vi "filter.vi"(0 "Image In":T2, 1 "Red BCG Values (Brightness 1)":T1={"Brightness"=142.42021, "Contrast"=69.80851, "Gamma"=2.51808}, 2 "Green BCG Values (Brightness 1)":T1={"Brightness"=142.42021, "Contrast"=69.80851, "Gamma"=2.51808}, 3 "Blue BCG Values (Brightness 1)":T1={"Brightness"=142.42021, "Contrast"=69.80851, "Gamma"=2.51808}, 4 "Range (Threshold 1)":cluster{"Lower value":sgl, "Upper value":sgl}={"Lower value"=109.28571, "Upper value"=255.0}, 7 "error in":errorcluster) -> (20 "Image Out":T2, 21 "Number of Particles (Particle Analysis 1)":i32, 22 "Particle Measurements (Pixels) (Particle Analysis 1)":dbl[][](array[numeric]) format="%.2f", 23 "Particle Measurements (Real-World) (Particle Analysis 1)":dbl[][](array[numeric]) format="%.2f", 27 "error out":errorcluster)   [LabVIEW 2020]
uses:
  <vilib>/vision/Image Controls.llb/IMAQ Image.ctl
  <vilib>/vision/NI_Vision_Development_Module.lvlib
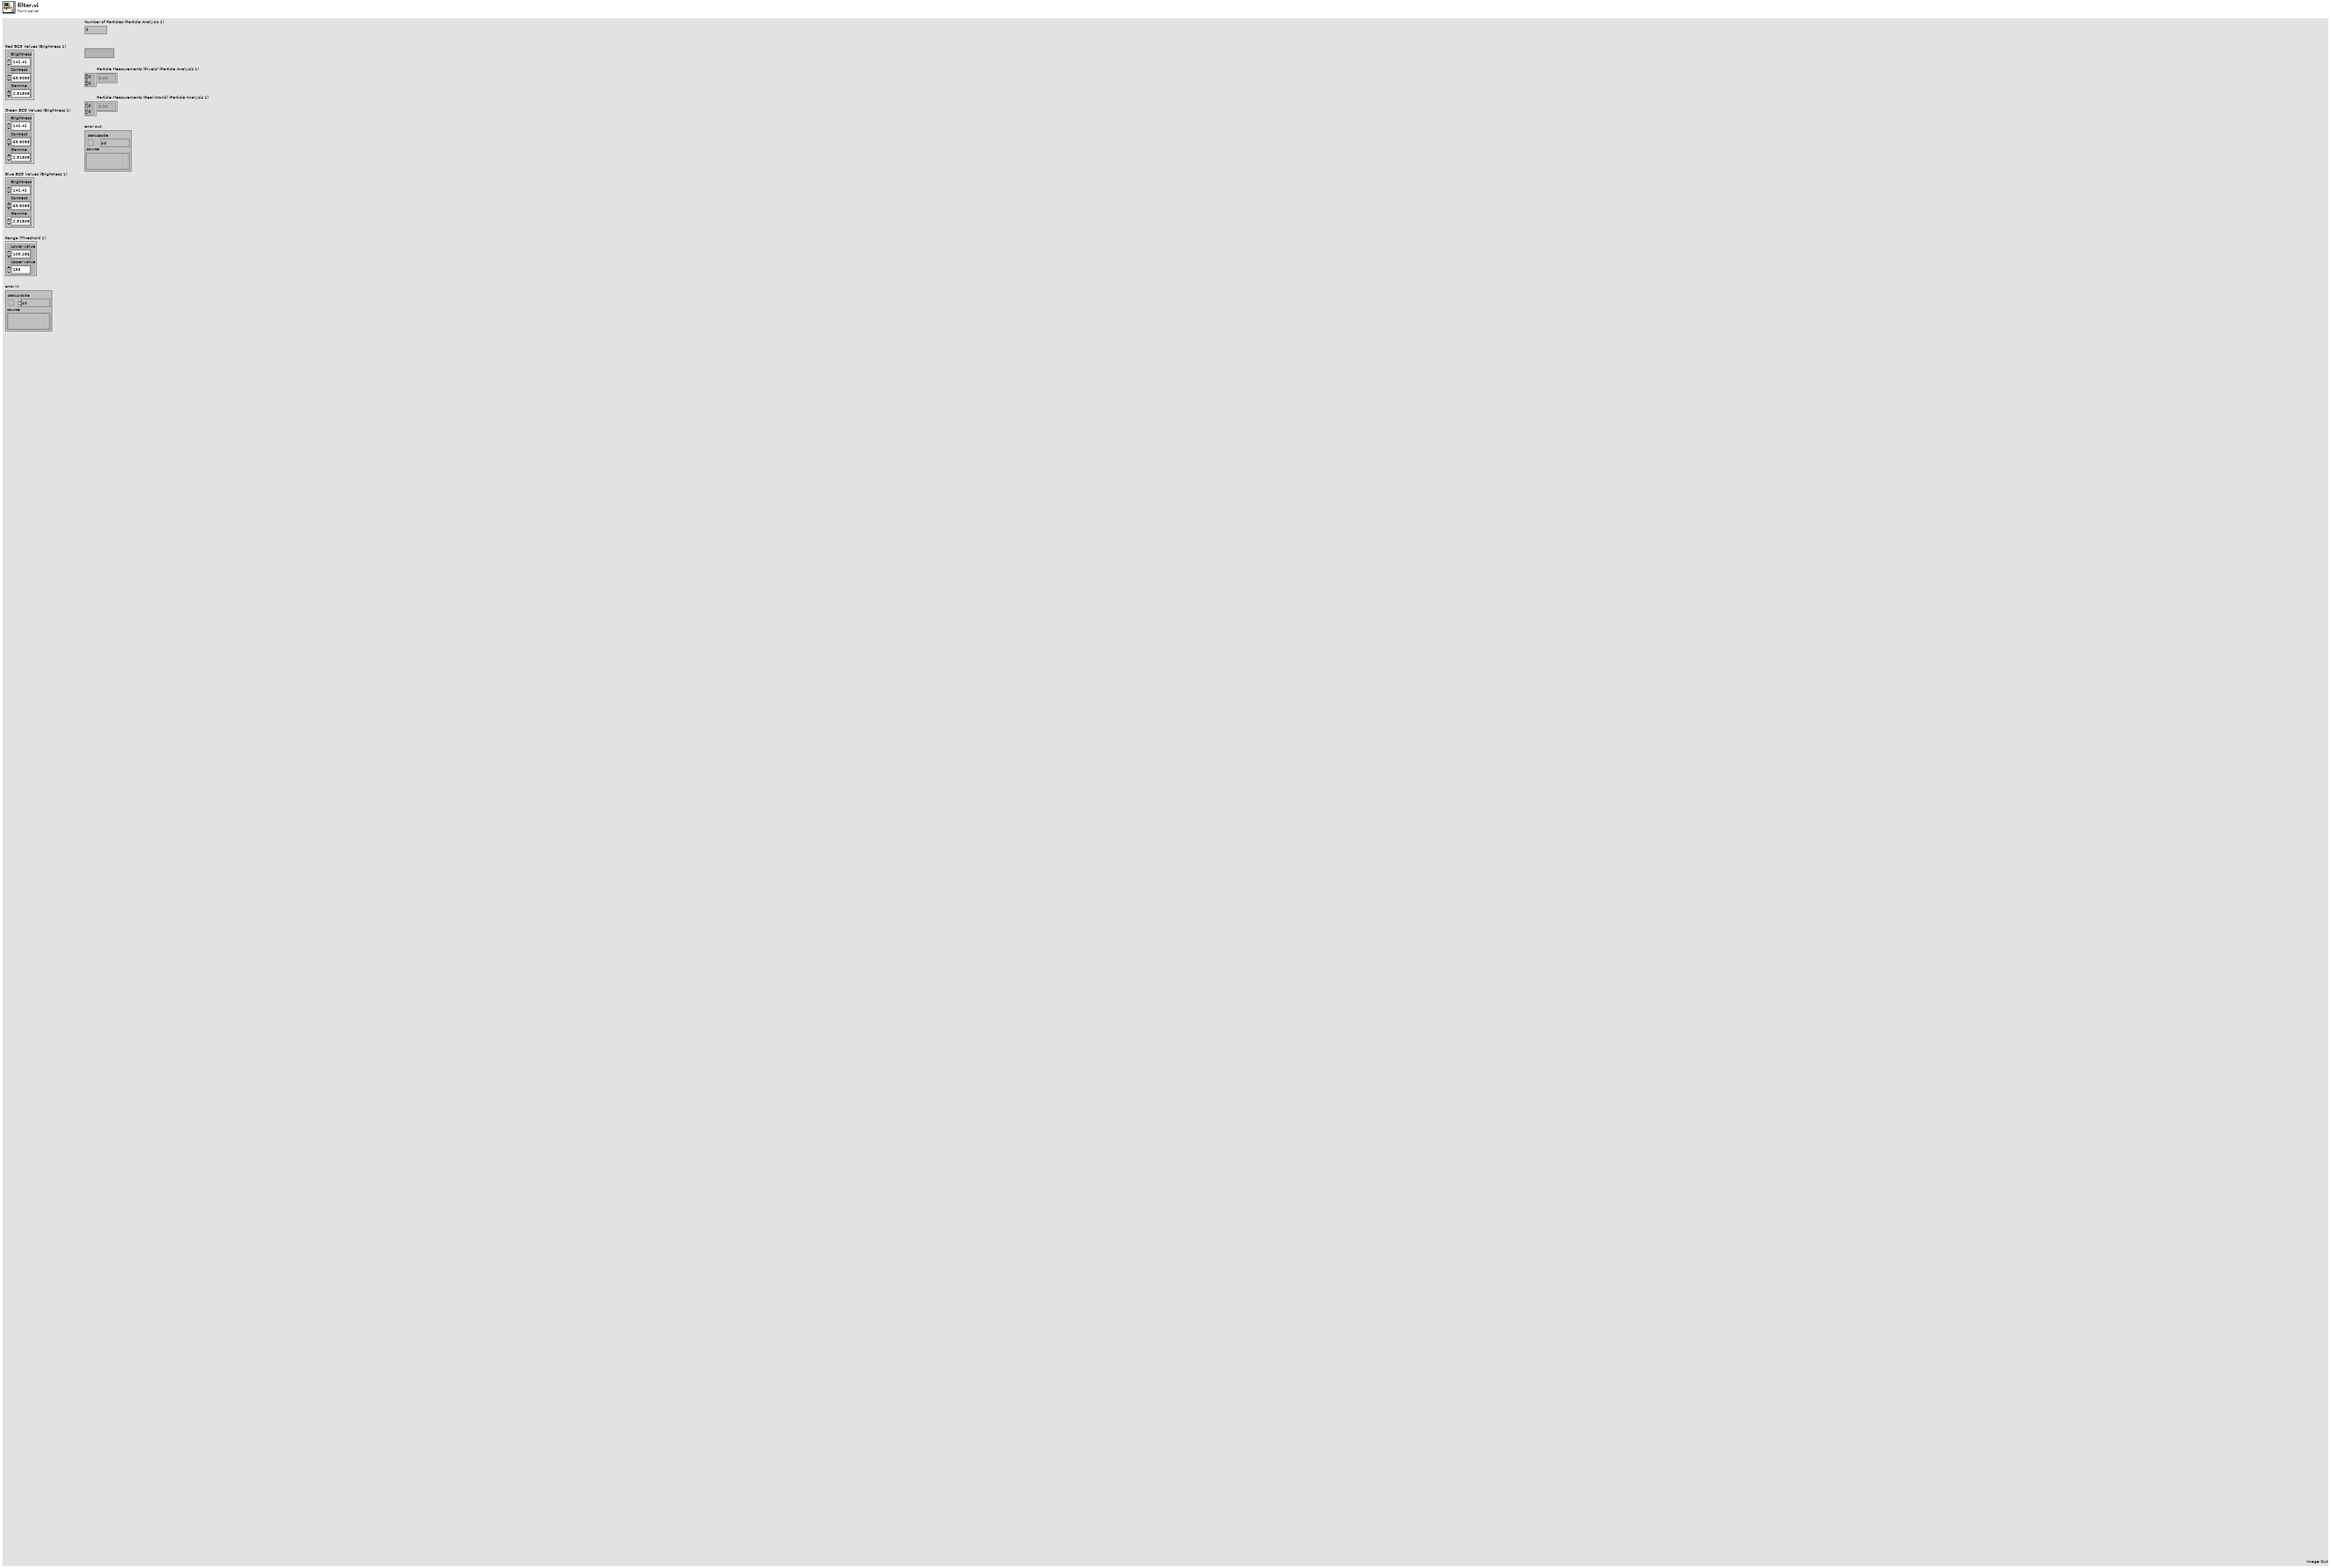
[diagram p1: front panel]
types:
  T1 = cluster{"Brightness":sgl, "Contrast":sgl, "Gamma":sgl}
  T2 = typedef "IMAQ Image.ctl" = refnum<image>
  T3 = cluster{"Measurement Parameter":i32, "Range Lower Value":dbl, "Range Upper Value":dbl, "Range":bool, "Measurement Type":bool}[]
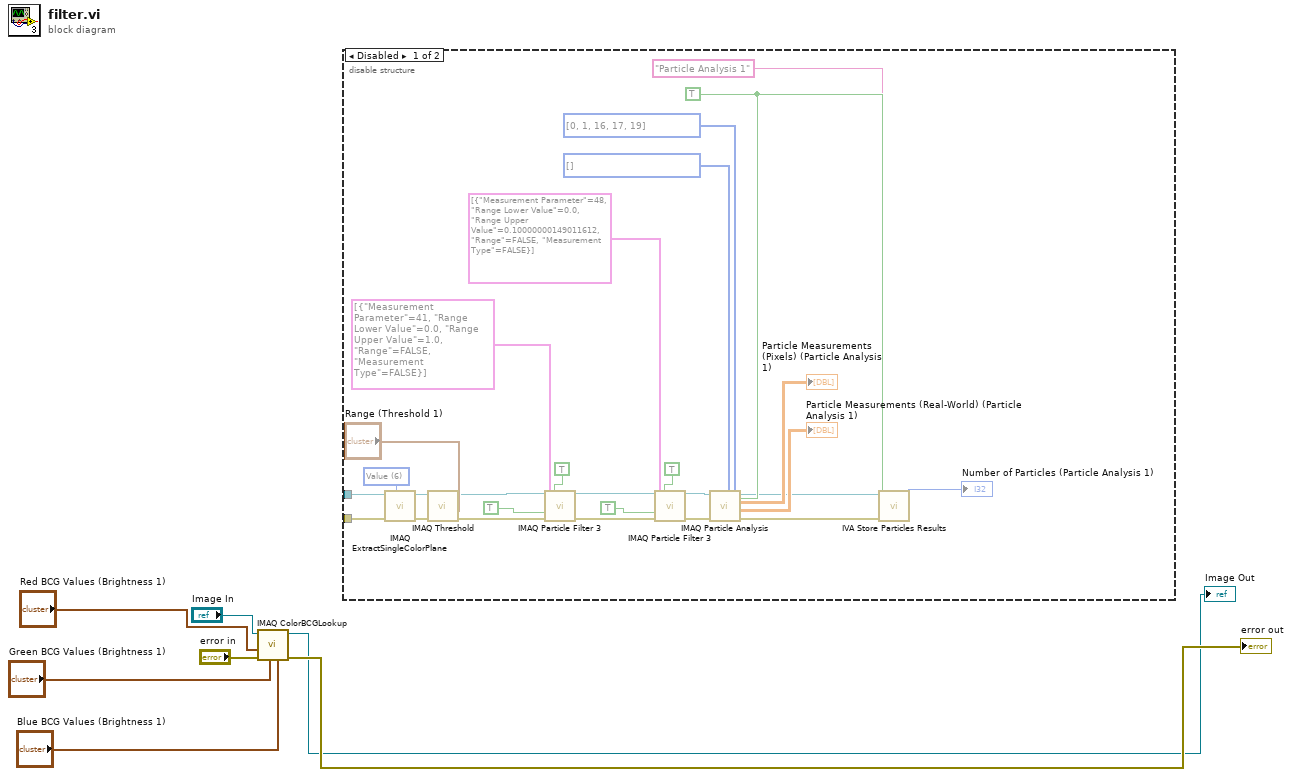
[diagram p0: block diagram]
diagram:
  n1 = call "IMAQ ColorBCGLookup"("Blue BCG Values"="Blue BCG Values (Brightness 1)", "Green BCG Values"="Green BCG Values (Brightness 1)", "error in (no error)"="error in", "Red BCG Values"="Red BCG Values (Brightness 1)", "Image Src"="Image In") -> ("error out"=→"error out":errorcluster, "Image Dst Out"=→"Image Out":T2)  [unwired: 2 in, 3 out]
  n2 = disable-structure shown="Disabled" {
    disable-tunnel: _ -> [w33 _]
    disable-tunnel: _ -> [w32 _]
    frame Disabled {
      w17 = i32[] [] items=["Center of Mass X", "Center of Mass Y", "First Pixel X", "First Pixel Y", "Bounding Rect Left", "Bounding Rect Top", "Bounding Rect Right", "Bounding Rect Bottom", "Max Feret Diameter Start X", "Max Feret Diameter Start Y", "Max Feret Diameter End X", "Max Feret Diameter End Y", "Max Horiz. Segment Length Left", "Max Horiz. Segment Length Right", "Max Horiz. Segment Length Row", "-", "Bounding Rect Width", "Bounding Rect Height", "Bounding Rect Diagonal", "Perimeter", "Convex Hull Perimeter", "Holes' Perimeter", "Max Feret Diameter", "Equivalent Ellipse Major Axis", "Equivalent Ellipse Minor Axis", "Equivalent Ellipse Minor Axis (Feret)", "Equivalent Rect Long Side", "Equivalent Rect Short Side", "Equivalent Rect Diagonal", "Equivalent Rect Short Side (Feret)", "Average Horiz. Segment Length", "Average Vert. Segment Length", "Hydraulic Radius", "Waddel Disk Diameter", "-", "Area", "Holes' Area", "Particle & Holes' Area", "Convex Hull Area", "Image Area", "-", "Number of Holes", "Number of Horiz. Segments", "Number of Vert. Segments", "-", "Orientation", "Max Feret Diameter Orientation", "-", "% Area/Image Area", "% Area/(Particle & Holes' Area)", "Ratio of Equivalent Ellipse Axes", "Ratio of Equivalent Rect Sides", "-", "Elongation Factor", "Compactness Factor", "Heywood Circularity Factor", "Type Factor", "-", "Sum X", "Sum Y", "Sum XX", "Sum XY", "Sum YY", "Sum XXX", "Sum XXY", "Sum XYY", "Sum YYY", "-", "Moment of Inertia XX", "Moment of Inertia XY", "Moment of Inertia YY", "Moment of Inertia XXX", "Moment of Inertia XXY", "Moment of Inertia XYY", "Moment of Inertia YYY", "Norm. Moment of Inertia XX", "Norm. Moment of Inertia XY", "Norm. Moment of Inertia YY", "Norm. Moment of Inertia XXX", "Norm. Moment of Inertia XXY", "Norm. Moment of Inertia XYY", "Norm. Moment of Inertia YYY", "Hu Moment 1", "Hu Moment 2", "Hu Moment 3", "Hu Moment 4", "Hu Moment 5", "Hu Moment 6", "Hu Moment 7"] ("Real-World Measurements")
      w18 = i32[] [0, 1, 16, 17, 19] items=["Center of Mass X", "Center of Mass Y", "First Pixel X", "First Pixel Y", "Bounding Rect Left", "Bounding Rect Top", "Bounding Rect Right", "Bounding Rect Bottom", "Max Feret Diameter Start X", "Max Feret Diameter Start Y", "Max Feret Diameter End X", "Max Feret Diameter End Y", "Max Horiz. Segment Length Left", "Max Horiz. Segment Length Right", "Max Horiz. Segment Length Row", "-", "Bounding Rect Width", "Bounding Rect Height", "Bounding Rect Diagonal", "Perimeter", "Convex Hull Perimeter", "Holes' Perimeter", "Max Feret Diameter", "Equivalent Ellipse Major Axis", "Equivalent Ellipse Minor Axis", "Equivalent Ellipse Minor Axis (Feret)", "Equivalent Rect Long Side", "Equivalent Rect Short Side", "Equivalent Rect Diagonal", "Equivalent Rect Short Side (Feret)", "Average Horiz. Segment Length", "Average Vert. Segment Length", "Hydraulic Radius", "Waddel Disk Diameter", "-", "Area", "Holes' Area", "Particle & Holes' Area", "Convex Hull Area", "Image Area", "-", "Number of Holes", "Number of Horiz. Segments", "Number of Vert. Segments", "-", "Orientation", "Max Feret Diameter Orientation", "-", "% Area/Image Area", "% Area/(Particle & Holes' Area)", "Ratio of Equivalent Ellipse Axes", "Ratio of Equivalent Rect Sides", "-", "Elongation Factor", "Compactness Factor", "Heywood Circularity Factor", "Type Factor", "-", "Sum X", "Sum Y", "Sum XX", "Sum XY", "Sum YY", "Sum XXX", "Sum XXY", "Sum XYY", "Sum YYY", "-", "Moment of Inertia XX", "Moment of Inertia XY", "Moment of Inertia YY", "Moment of Inertia XXX", "Moment of Inertia XXY", "Moment of Inertia XYY", "Moment of Inertia YYY", "Norm. Moment of Inertia XX", "Norm. Moment of Inertia XY", "Norm. Moment of Inertia YY", "Norm. Moment of Inertia XXX", "Norm. Moment of Inertia XXY", "Norm. Moment of Inertia XYY", "Norm. Moment of Inertia YYY", "Hu Moment 1", "Hu Moment 2", "Hu Moment 3", "Hu Moment 4", "Hu Moment 5", "Hu Moment 6", "Hu Moment 7"] ("Pixel Measurements")
      w12 = TRUE ("Connectivity 4/8 (8)")
      w34 = 6 items=["Red", "Green", "Blue", "Hue", "Saturation", "Luminance", "Value", "Intensity"] ("Color Plane")
      n3 = call "IMAQ ExtractSingleColorPlane"("Color Plane"=w34, "error in (no error)"=w32, "Image Src"=w33) -> ("error out"=w29:errorcluster, "Image Dst Out"=w30:T2)  [unwired: 1 in, 6 out]
      n4 = call "IMAQ Threshold"("error in (no error)"=w29, "Range"="Range (Threshold 1)", "Image Src"=w30) -> ("error out"=w25:errorcluster, "Image Dst Out"=w26:T2)  [unwired: 3 in, 4 out]
      n5 = call "IMAQ Particle Filter 3"("Image Src"=w26, "Connectivity 4/8 (8)"=TRUE, "Selection Values"=T3 [{"Measurement Parameter"=41, "Range Lower Value"=0.0, "Range Upper Value"=1.0, "Range"=FALSE, "Measurement Type"=FALSE}], "Keep/Remove Particles (F)"=TRUE ("Keep/Remove Particles"), "error in (no error)"=w25) -> ("Image Dst Out"=w21:T2, "error out"=w20:errorcluster)  [unwired: 4 in, 5 out]
      n6 = call "IMAQ Particle Filter 3"("Image Src"=w21, "Connectivity 4/8 (8)"=TRUE, "Selection Values"=T3 [{"Measurement Parameter"=48, "Range Lower Value"=0.0, "Range Upper Value"=0.10000000149011612, "Range"=FALSE, "Measurement Type"=FALSE}], "Keep/Remove Particles (F)"=TRUE ("Keep/Remove Particles"), "error in (no error)"=w20) -> ("Image Dst Out"=w13:T2, "error out"=w14:errorcluster)  [unwired: 4 in, 5 out]
      n7 = call "IMAQ Particle Analysis"("Connectivity 4/8 (8)"=w12, "error in (no error)"=w14, "Real-World Measurements"=w17, "Pixel Measurements"=w18, "Image"=w13) -> ("error out"=w9:errorcluster, "Particle Measurements (Real-World)"=→"Particle Measurements (Real-World) (Particle Analysis 1)":dbl[][], "Particle Measurements (Pixels)"=→"Particle Measurements (Pixels) (Particle Analysis 1)":dbl[][], "Image Out (duplicate)"=w11:T2)  [unwired: 3 out]
      n8 = call <vilib>:"IVA Store Particles Results.vi"("error in (no error)"=w9, "Connectivity 4/8 (8)"=w12, "Step Name"="Particle Analysis 1", "Image in"=w11) -> ("Number of Particles"=→"Number of Particles (Particle Analysis 1)":i32)  [unwired: 7 out]
    }
    frame Enabled {
    }
  }
